vi "SVT SINAD.vi"   [LabVIEW 2017, in "SoundVib_Distortion.lvlib"]
doc: "Performs a signal in noise and distortion (SINAD) analysis, including measuring the fundamental tone, and returns the detected fundamental frequency, detected fundamental amplitude, and SINAD level in dB. Total harmonic distortion plus noise (THD + N) is the negative of SINAD in dB. Wire data to the <B>scaled signal [EU]</B> input to determine the polymorphic instance to use or manually select the instance.\n\nThe following formula calculates SINAD:\n\nSINAD = sqrt(F^2 + N^2 + H^2) / sqrt(H^2 + N^2)\n\nwhere F is the fundamental tone RMS level, N is the noise RMS level, and H is the harmonic RMS level."
uses:
  <vilib>/addons/Sound and Vibration/svt_Distortion/SoundVib_Distortion.lvlib
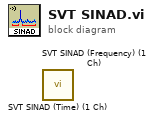
[diagram p0: block diagram]
diagram:
  n1 = call <vilib>:"SVT SINAD (Time) (1 Ch).vi"() -> ()  [unwired: 14 in, 6 out]
  n2 = call <vilib>:"SVT SINAD (Frequency) (1 Ch).vi"() -> ()  [unwired: 14 in, 6 out]
